vi "Read A.vi"(8 "error in (no error)":errorcluster, 11 "Math Operations in":refnum<class "Math Operations.lvclass">) -> (0 "error out":errorcluster, 2 "A":dbl, 3 "Math Operations out":refnum<class "Math Operations.lvclass">)   [LabVIEW 2020, in "Math Operations.lvclass"]
uses:
  Math Operations.lvclass
  Math Operations.lvclass/Math Operations.ctl
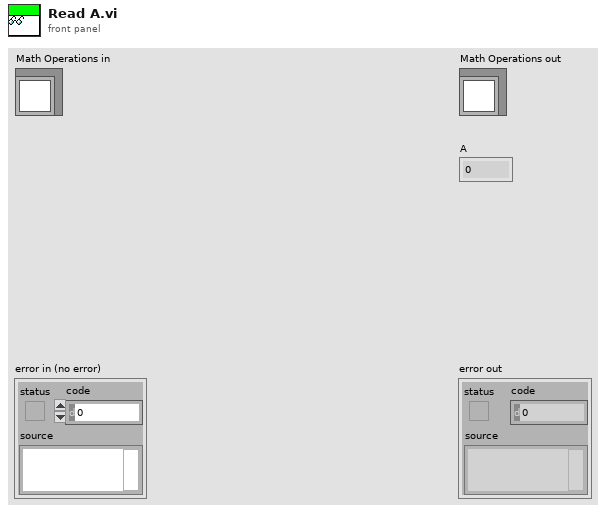
[diagram p1: front panel]
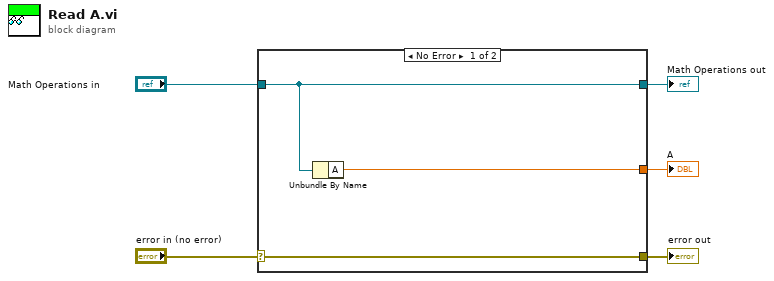
[diagram p0: block diagram]
diagram:
  n1 = case shown="No Error" "error in (no error)" {
    selector: "error in (no error)" -> [w8 w9]
    tunnel: [w8 w9] -> w4
    tunnel: [w7 w10] -> w2
    tunnel: "Math Operations in" -> [w7 w10]
    tunnel: [w6 _] -> w1
    frame No Error {
      n2 = Unbundle By Name(w7) -> ("A"=w6:dbl)
    }
    frame Error {
    }
  }
  "error out" <- w4
  "Math Operations out" <- w2
  "A" <- w1
